vi "clicked_trajectory.vi"(8 "error in (no error)":errorcluster, 11 "TrajectoryTS090820Circular2D in":refnum<class "TrajectoryTS090820Circular2D.lvclass">) -> (0 "error out":errorcluster, 3 "TrajectoryTS090820Circular2D out":refnum<class "TrajectoryTS090820Circular2D.lvclass">)   [LabVIEW 2010, in "TrajectoryTS090820Circular2D.lvclass"]
uses:
  TrajectoryTS090820Circular2D.lvclass
  TrajectoryTS090820Circular2D.lvclass/TrajectoryTS090820Circular2D.ctl
  common/classes/Image/Image/Image.lvclass
  <vilib>/express/express arith-compare/Formula/XNode/ExpressFormulaBlockNode.xnode
  <vilib>/Analysis/BLAS.llb/dnrm2 - Vector 2-Norm (DBL).vi
  <vilib>/Analysis/baseanly.llb/Real Dot Product.vi
  <vilib>/Analysis/NI_AALBLAS.lvlib
  <vilib>/Analysis/NI_AALBase.lvlib
panel:
  in  "clicked points":i32[][](array[numeric])
  in  "circular trajectory":bool=TRUE
  in  "Numeric":i32
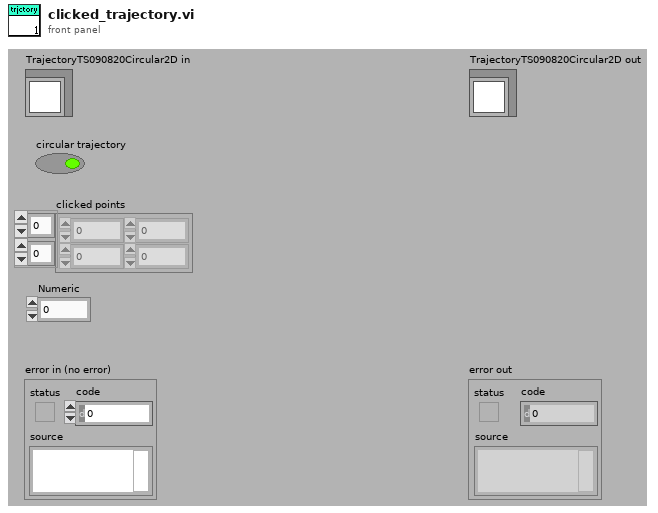
[diagram p1: front panel]
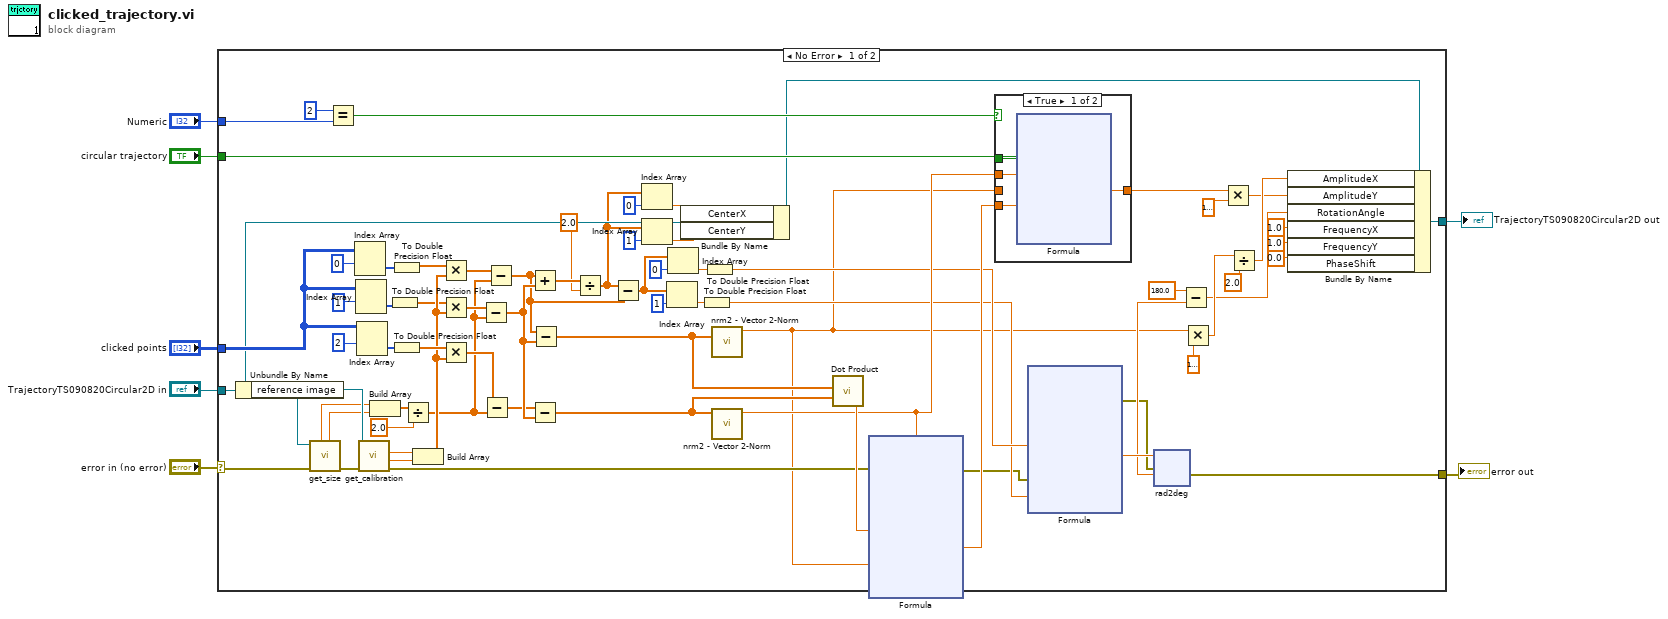
[diagram p0: block diagram]
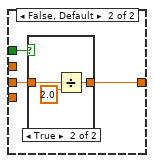
[diagram p2: hidden frame]
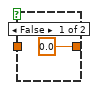
[diagram p3: hidden frame]
diagram:
  n1 = case shown="No Error" "error in (no error)" {
    selector: "error in (no error)" -> [w28 w131]
    tunnel: [w10 w131] -> w1
    tunnel: [w59 w130] -> w2
    tunnel: "TrajectoryTS090820Circular2D in" -> [w32 w130]
    tunnel: "clicked points" -> [w43 _]
    tunnel: "Numeric" -> [w73 _]
    tunnel: "circular trajectory" -> [w74 _]
    frame No Error {
      n2 = Unbundle By Name(w32) -> ("reference image"=w26:refnum<class "Image.lvclass">)
      n3 = call-dynamic "get_size.vi"("error in (no error)"=w28, "Image in"=w26) -> ("error out"=w27:errorcluster, "physical size y"=w24:dbl, "physical size x"=w25:dbl)  [unwired: 2 in, 5 out]
      n4 = Equal?(x=2, y=w73) -> (x = y?=w78:bool)
      n5 = Index Array(array=w43, index (row)=0 ("disabled index (col)")) -> (element=w42:i32[])  [unwired: 1 in]
      n6 = Index Array(array=w43, index (row)=1 ("disabled index (col)")) -> (element=w41:i32[])  [unwired: 1 in]
      n7 = Index Array(array=w43, index (row)=2 ("disabled index (col)")) -> (element=w40:i32[])  [unwired: 1 in]
      n8 = call "get_calibration.vi"("error in (no error)"=w27, "Image.lvclass in"=w26) -> ("error out"=w31:errorcluster, "y"=w29:dbl, "x"=w30:dbl)  [unwired: 2 in, 5 out]
      n9 = Build Array(w25, w24) -> (w17:dbl[])
      n10 = To Double Precision Float(number=w41) -> (double precision float=w34:dbl[])
      n11 = To Double Precision Float(number=w42) -> (double precision float=w33:dbl[])
      n12 = To Double Precision Float(number=w40) -> (double precision float=w36:dbl[])
      n13 = Divide(x=w17, y=2.0 ("physical size y")) -> (x/y=w16:dbl[])
      n14 = Build Array(w30, w29) -> (w35:dbl[])
      n15 = Multiply(x=w33, y=w35) -> (x*y=w21:dbl[])
      n16 = Multiply(x=w34, y=w35) -> (x*y=w23:dbl[])
      n17 = Multiply(x=w36, y=w35) -> (x*y=w19:dbl[])
      n18 = Subtract(x=w23, y=w16) -> (x-y=w22:dbl[])
      n19 = Subtract(x=w19, y=w16) -> (x-y=w18:dbl[])
      n20 = Subtract(x=w21, y=w16) -> (x-y=w20:dbl[])
      n21 = Add(x=w20, y=w22) -> (x+y=w39:dbl[])
      n22 = Subtract(x=w18, y=w22) -> (x-y=w37:dbl[])
      n23 = Subtract(x=w20, y=w22) -> (x-y=w38:dbl[])
      n24 = Divide(x=w39, y=2.0 ("Horizontal")) -> (x/y=w13:dbl[])
      n25 = Subtract(x=w13, y=w20) -> (x-y=w56:dbl[])
      n26 = Index Array(array=w13, index=0 ("disabled index (col)")) -> (element=w63:dbl)
      n27 = Index Array(array=w13, index=1 ("disabled index (col)")) -> (element=w61:dbl)
      n28 = Index Array(array=w56, index=1) -> (element=w53:dbl)
      n29 = Index Array(array=w56, index=0) -> (element=w55:dbl)
      n30 = Bundle By Name(cluster=w32, "CenterX"=w63, "CenterY"=w61) -> (w60:refnum<class "TrajectoryTS090820Circular2D.lvclass">)
      n31 = To Double Precision Float(number=w53) -> (double precision float=w52:dbl)
      n32 = To Double Precision Float(number=w55) -> (double precision float=w54:dbl)
      n33 = call-poly <vilib>:"nrm2 - Vector 2-Norm.vi"("x"=w38) -> ("dnrm2"=w9:dbl)  [unwired: 9 in, 1 out]
      n34 = call-poly <vilib>:"nrm2 - Vector 2-Norm.vi"("x"=w37) -> ("dnrm2"=w76:dbl)  [unwired: 9 in, 1 out]
      n35 = call-poly <vilib>:"Dot Product.vi"("Y Vector"=w37, "X Vector"=w38) -> ("X * Y"=w77:dbl)  [unwired: 1 out]
      n36 = xnode "Formula"("dot_u_v"=w77, "u"=w9, "v"=w76, "error in (no error)"=w31) -> ("Result"=w75:dbl, "error out"=w12:errorcluster)
      n37 = case shown="True" w78 {
        tunnel: w76 -> [w112 _]
        tunnel: w75 -> [w111 _]
        tunnel: [w110 w125] -> w71
        tunnel: w74 -> [_ w124]
        tunnel: w9 -> [_ w123]
        frame True {
          n38 = xnode "Formula"("a"=w112, "alfa"=w111) -> ("Result"=w110:dbl)  [unwired: 1 in, 1 out]
        }
        frame False, Default {
          n39 = case shown="True" w124 {
            tunnel: [0.0 ("Result") w127] -> w125
            tunnel: w123 -> [_ w128]
            frame False {
            }
            frame True {
              n40 = Divide(x=w128, y=2.0) -> (x/y=w127:dbl)
            }
          }
        }
      }
      n41 = xnode "Formula"("x"=w54, "error in (no error)"=w12, "y"=w52) -> ("Result"=w50:dbl, "error out"=w11:errorcluster)
      n42 = xnode "rad2deg"("alfa"=w50, "error in (no error)"=w11) -> ("Result"=w49:dbl, "error out"=w10:errorcluster)
      n43 = Subtract(x=180.0 ("y"), y=w49) -> (x-y=w44:dbl)
      n44 = Multiply(x=w9, y=dbl[unit] 1e-06 ("dimension size")) -> (x*y=w67:dbl[unit])
      n45 = Multiply(x=w71, y=dbl[unit] 1e-06 ("dimension size")) -> (x*y=w45:dbl[unit])
      n46 = Divide(x=w67, y=2.0) -> (x/y=w65:dbl[unit])
      n47 = Bundle By Name(cluster=w60, "AmplitudeX"=w65, "AmplitudeY"=w45, "RotationAngle"=w44, "FrequencyX"=1.0 ("settings.x frequency"), "FrequencyY"=1.0 ("settings.y frequency"), "PhaseShift"=0.0 ("settings.phase shift")) -> (w59:refnum<class "TrajectoryTS090820Circular2D.lvclass">)
    }
    frame Error {
    }
  }
  "error out" <- w1
  "TrajectoryTS090820Circular2D out" <- w2
